vi "AddDataToPlots.vi"(0 "Scope5761 in":refnum<class "Scope5782_six_channel.lvclass">, 1 "Display":T4, 2 "Buffer":T3, 3 "Unwrap phase":bool, 4 "Transfer speed":T6, 5 "Reference for phase":T7, 6 "Window":T2=1 items=["Rectangle"=0, "Hanning"=1, "Hamming"=2, "Blackman-Harris"=3, "Exact Blackman"=4, "Blackman"=5, "Flat Top"=6, "4 Term B-Harris "=7, "7 Term B-Harris"=8, "Low Sidelobe"=9, "Blackman Nuttall"=11, "Triangle"=30, "Bartlett-Hanning"=31, "Bohman"=32, "Parzen"=33, "Welch"=34, "Kaiser"=60, "Dolph-Chebyshev"=61, "Gaussian"=62], 7 "Unit":T5, 9 "#bins":i32=1 min=1 max=16, 10 "Phase/s":dbl, 11 "Update once lower":refnum<vi>, 13 "Update once upper":refnum<vi>) -> (17 "Uppder data":dbl[][](array[numeric]), 18 "magnitude out":cluster{"f0":dbl, "df":dbl, "magnitude":dbl[]}, 19 "Lower data":dbl[][](array[numeric]), 20 "Scope5761 out":refnum<class "Scope5782_six_channel.lvclass">, 21 "Freqdata":cluster{"f0":dbl, "df":dbl, "magnitude":dbl[]}[](array[cluster]), 22 "Any read?":bool, 23 "Write upper":T1, 25 "Write lower":T1)   [LabVIEW 2018]
uses:
  controls/Channel_select_2fpga.ctl
  controls/host_transfer_speed.ctl
  controls/power_spectrum_unit.ctl
  controls/Data_calc_mode.ctl
  controls/Data_display_mode.ctl
  <vilib>/Analysis/4window.llb/windowTd.ctl
  Scope5782_six_channel/Scope5782_six_channel.lvclass
  C:/PXIe/InProgress/source2/Host/Scope/ScopeBase/ScopeBase.lvclass
  controls/PlotUpdate type.ctl
  Scope5782_six_channel/Scope5782_six_channel.lvclass/Scope5782_six_channel.ctl
  ScopeBase/ScopeBase.lvclass/ScopeBase.ctl
  ScopeBase/ScopeBase.lvclass
  <vilib>/Analysis/NI_AALPro.lvlib
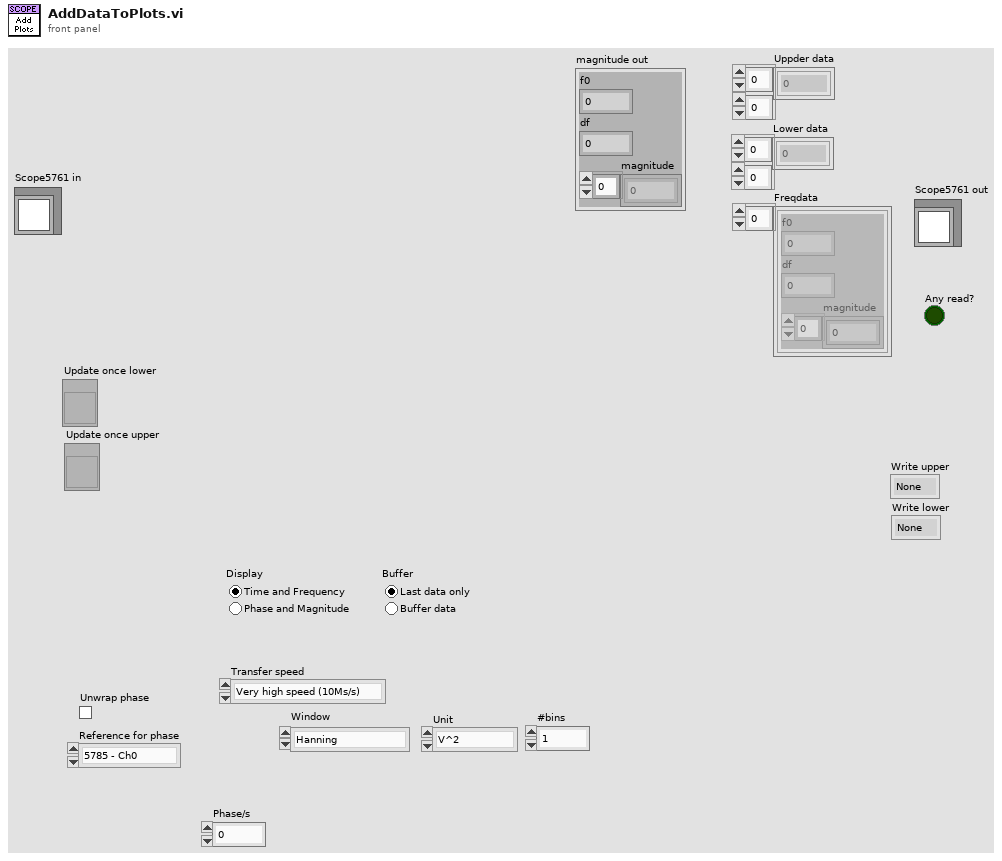
[diagram p1: front panel]
types:
  T1 = typedef "PlotUpdate type.ctl" = enum16{"None", "Graph", "Chart", "Freq"}
  T2 = typedef "NI_AALPro.lvlib/windowTd.ctl" = u32
  T3 = typedef "Data_display_mode.ctl" = enum32{"Last data only", "Buffer data"}
  T4 = typedef "Data_calc_mode.ctl" = enum32{"Time and Frequency", "Phase and Magnitude"}
  T5 = typedef "power_spectrum_unit.ctl" = enum16{"V^2", "V", "dBV"}
  T6 = typedef "host_transfer_speed.ctl" = enum16{"Very high speed (10Ms/s)", "High speed (1Ms/s)", "Low speed (50kS/s)", "Ultra low speed (20kS/s)"}
  T7 = typedef "Channel_select_2fpga.ctl" = enum16{"5785 - Ch0", "5785 - Ch1 cavity", "5785 - Ch1", "5761 - Ch0", "5761 - Ch1", "5761 - Ch2", "5761 - Ch3", "Fixed"}
  T8 = typedef "ScopeMode.ctl" = enum16{"Stopped", "Single", "Running", "Continuous"}
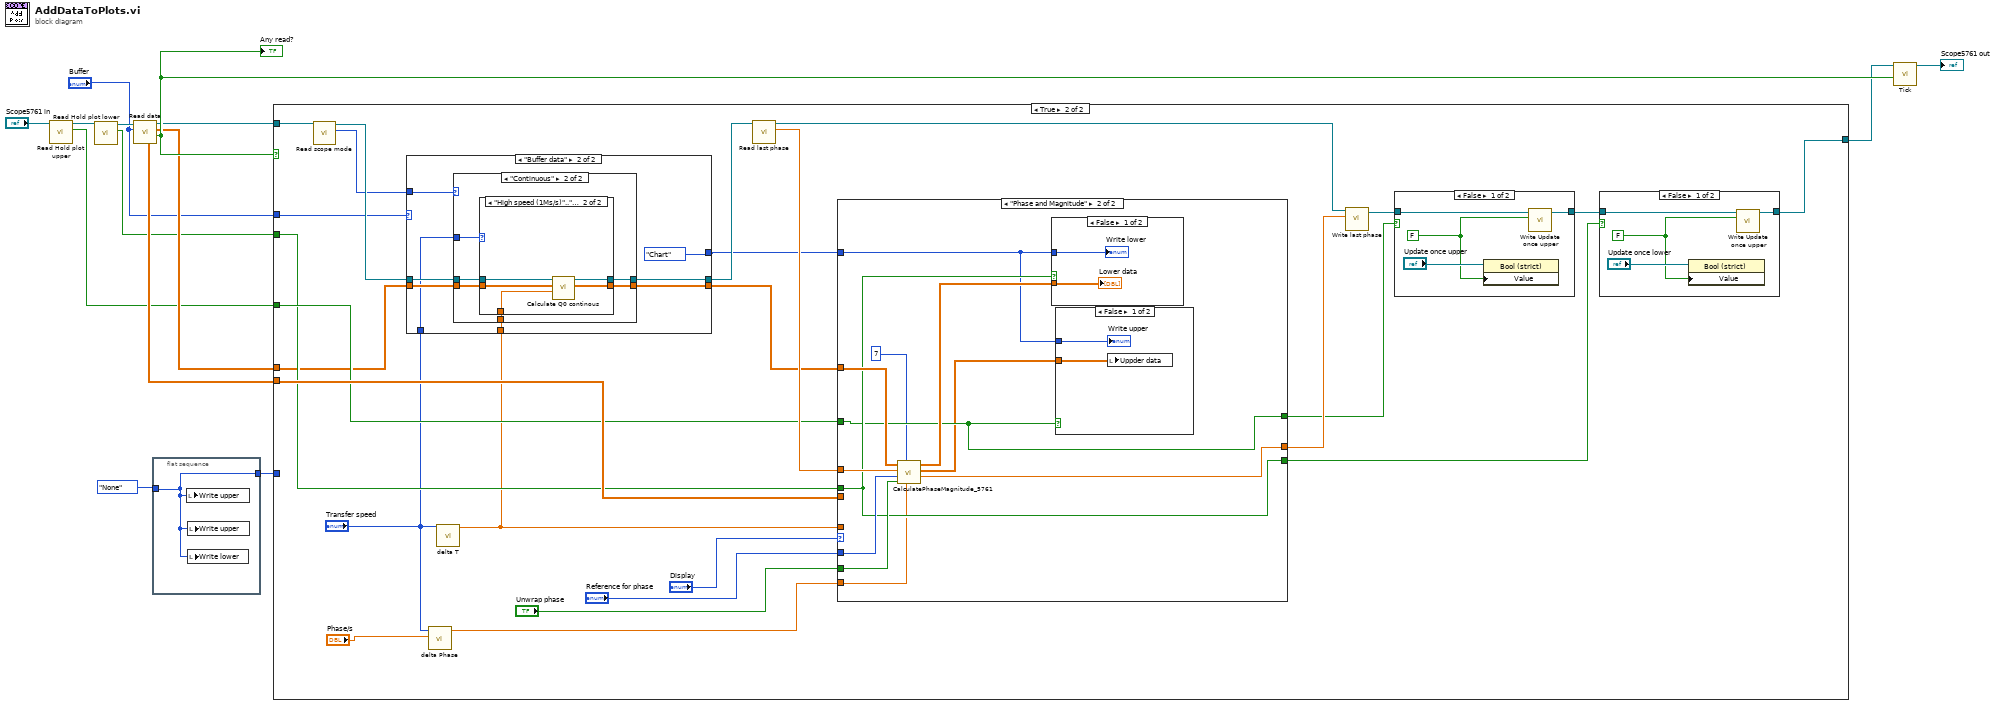
[diagram p0: block diagram]
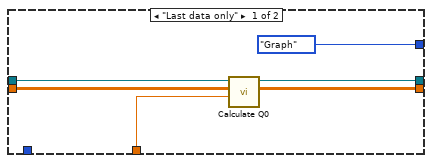
[diagram p3: hidden frame]
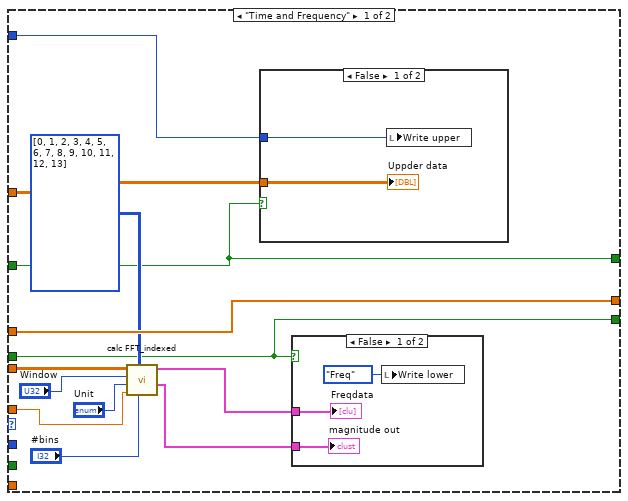
[diagram p8: hidden frame]
diagram:
  n1 = call "Read Hold plot upper.vi"("Scope5761"="Scope5761 in") -> ("Hold plot upper"=w9:bool, "Scope5761"=w11:refnum<class "Scope5782_six_channel.lvclass">)  [unwired: 8 in, 1 out]
  n2 = call "Read Hold plot lower.vi"("Scope5761"=w11) -> ("Hold plot lower"=w8:bool, "Scope5761"=w10:refnum<class "Scope5782_six_channel.lvclass">)  [unwired: 8 in, 1 out]
  n3 = call-dynamic "Read data.vi"("Buffer mode"="Buffer", "Scope5785_six_channel"=w10) -> ("Any read?"=w14:bool, "Data"=w13:dbl[][], "Scope5785_six_channel out"=w7:refnum<class "Scope5782_six_channel.lvclass">, "FFT buffer"=w12:dbl[][])  [unwired: 5 in, 1 out]
  "Any read?" <- w14
  n4 = flat-sequence {
    tunnel: PlotUpdate_type."None" ("Write upper") -> [w15]
    tunnel: [w15] -> w2
    frame #0 {
      n5 = local write "Write upper"(w15) -> ()
      n6 = local write "Write upper"(w15) -> ()
      n7 = local write "Write lower"(w15) -> ()
    }
  }
  n8 = case shown="True" w14 {
    tunnel: w13 -> [_ w21]
    tunnel: w12 -> [_ w42]
    tunnel: w9 -> [_ w39]
    tunnel: w8 -> [_ w38]
    tunnel: "Buffer" -> [_ w23]
    tunnel: [w16 w32] -> w6
    tunnel: w7 -> [w16 w26]
    tunnel: w2 -> [_ _]
    frame False {
    }
    frame True {
      n9 = call "Read scope mode.vi"("ScopeBase in"=w26) -> ("scope mode"=w27:T8, "ScopeBase out"=w28:refnum<class "Scope5782_six_channel.lvclass">)  [unwired: 8 in, 1 out]
      n10 = call "delta Phase.vi"("Phase/s [kHz]"="Phase/s", "Tranfer speed"="Transfer speed") -> ("phase per sample (rad)"=w18:dbl)  [unwired: 9 in]
      n11 = call "delta T.vi"("Tranfer speed"="Transfer speed") -> ("dt"=w22:dbl)  [unwired: 10 in]
      n12 = case shown="\"Buffer data\"" w23 {
        tunnel: [PlotUpdate_type."Graph" ("Write upper") PlotUpdate_type."Chart" ("Write upper")] -> w24
        tunnel: w22 -> [w47 w49]
        tunnel: w21 -> [w46 w52]
        tunnel: w28 -> [w45 w53]
        tunnel: [w44 w54] -> w25
        tunnel: [w43 w51] -> w20
        tunnel: w27 -> [_ w55]
        tunnel: "Transfer speed" -> [_ w50]
        frame "Last data only" {
          n13 = call "Calculate Q0.vi"("dt"=w47, "Data"=w46, "Scope5761 in"=w45) -> ("Data out"=w43:dbl[][], "Scope5761out"=w44:refnum<class "Scope5782_six_channel.lvclass">)  [unwired: 6 in, 1 out]
        }
        frame "Buffer data" {
          n14 = case shown="\"Continuous\"" w55 {
            tunnel: [w58 w62] -> w54
            tunnel: w53 -> [w58 w63]
            tunnel: w52 -> [w57 w61]
            tunnel: [w57 w60] -> w51
            tunnel: w50 -> [_ w64]
            tunnel: w49 -> [_ w59]
            frame "Stopped", Default {
            }
            frame "Continuous" {
              n15 = case shown="\"High speed (1Ms/s)\"..\"Ultra low speed (20kS/s)\"" w64 {
                tunnel: w63 -> [w66 w71]
                tunnel: [w66 w70] -> w62
                tunnel: w61 -> [w65 w69]
                tunnel: [w65 w68] -> w60
                tunnel: w59 -> [_ w67]
                frame "Very high speed (10Ms/s)", Default {
                }
                frame "High speed (1Ms/s)".."Ultra low speed (20kS/s)" {
                  n16 = call "Calculate Q0 continous.vi"("dt"=w67, "Data"=w69, "Scope5761 in"=w71) -> ("Data out"=w68:dbl[][], "Scope5761out"=w70:refnum<class "Scope5782_six_channel.lvclass">)  [unwired: 6 in, 1 out]
                }
              }
            }
          }
        }
      }
      n17 = call "Read last phase.vi"("ScopeBase in"=w25) -> ("last phase"=w40:dbl[], "ScopeBase out"=w31:refnum<class "Scope5782_six_channel.lvclass">)  [unwired: 8 in, 1 out]
      n18 = case shown="\"Phase and Magnitude\"" "Display" {
        tunnel: w42 -> [w91 _]
        tunnel: "Reference for phase" -> [_ w110]
        tunnel: w40 -> [w93 w109]
        tunnel: [w93 w108] -> w41
        tunnel: w22 -> [w92 _]
        tunnel: "Unwrap phase" -> [_ w107]
        tunnel: w20 -> [w90 w106]
        tunnel: w39 -> [w84 w104]
        tunnel: w38 -> [w85 w105]
        tunnel: [w85 w105] -> w29
        tunnel: [w84 w104] -> w30
        tunnel: w24 -> [w83 w102]
        tunnel: w18 -> [_ w100]
        frame "Time and Frequency" {
          n19 = call "calc FFT_indexed.vi"("#bins"="#bins", "IQ indexes"=i32[][] [[0, 1], [2, 3], [4, 5], [6, 7], [8, 9], [10, 11], [12, 13]], "dt"=w92, "Unit"="Unit", "Window"="Window", "data"=w91) -> ("magnitude out"=w82:cluster{"f0":dbl, "df":dbl, "magnitude":dbl[]}, "Power Spectrum / PSD"=w94:cluster{"f0":dbl, "df":dbl, "magnitude":dbl[]}[])  [unwired: 4 in]
          n20 = case shown="False" w84 {
            tunnel: w90 -> [w99 _]
            tunnel: w83 -> [w98 _]
            frame False {
              n21 = local write "Write upper"(w98) -> ()
              "Uppder data" <- w99
            }
            frame True {
            }
          }
          n22 = case shown="False" w85 {
            tunnel: w94 -> [w97 _]
            tunnel: w82 -> [w95 _]
            frame False {
              n23 = local write "Write lower"(PlotUpdate_type."Freq" ("Write lower")) -> ()
              "Freqdata" <- w97
              "magnitude out" <- w95
            }
            frame True {
            }
          }
        }
        frame "Phase and Magnitude" {
          n24 = call "CalculatePhaseMagnitude_5761.vi"("phase per sample (rad)"=w100, "Max num channels"=7, "unwrap phase"=w107, "phase reference channel"=w110, "previous phase"=w109, "data"=w106) -> ("last phase"=w108:dbl[], "Magnitude"=w103:dbl[][], "Phase"=w111:dbl[][])  [unwired: 3 in]
          n25 = case shown="False" w105 {
            tunnel: w111 -> [w115 _]
            tunnel: w102 -> [w114 _]
            frame False {
              "Lower data" <- w115
              "Write lower" <- w114
            }
            frame True {
            }
          }
          n26 = case shown="False" w104 {
            tunnel: w103 -> [w113 _]
            tunnel: w102 -> [w112 _]
            frame False {
              n27 = local write "Uppder data"(w113) -> ()
              "Write upper" <- w112
            }
            frame True {
            }
          }
        }
      }
      n28 = call "Write last phase.vi"("last phase"=w41, "ScopeBase in"=w31) -> ("ScopeBase out"=w34:refnum<class "Scope5782_six_channel.lvclass">)  [unwired: 8 in, 1 out]
      n29 = case shown="False" w30 {
        tunnel: w34 -> [w80 w81]
        tunnel: [w79 w81] -> w33
        frame False {
          w77 = FALSE ("Update once upper")
          n30 = property class="Bool (strict)"(reference="Update once upper", "Value"=w77) -> ()  [unwired: 1 in, 2 out]
          n31 = call "Write Update once upper.vi"("Update once upper"=w77, "Scope5761"=w80) -> ("Scope5761"=w79:refnum<class "Scope5782_six_channel.lvclass">)  [unwired: 8 in, 1 out]
        }
        frame True {
        }
      }
      n32 = case shown="False" w29 {
        tunnel: w33 -> [w73 w76]
        tunnel: [w74 w76] -> w32
        frame False {
          w72 = FALSE ("Update once upper")
          n33 = property class="Bool (strict)"(reference="Update once lower", "Value"=w72) -> ()  [unwired: 1 in, 2 out]
          n34 = call "Write Update once upper.vi"("Update once upper"=w72, "Scope5761"=w73) -> ("Scope5761"=w74:refnum<class "Scope5782_six_channel.lvclass">)  [unwired: 8 in, 1 out]
        }
        frame True {
        }
      }
    }
  }
  n35 = call "Tick.vi"("Any elements read?"=w14, "ScopeBase in"=w6) -> ("ScopeBase out"=→"Scope5761 out":refnum<class "Scope5782_six_channel.lvclass">)  [unwired: 8 in, 1 out]
